vi "XL320_Reset.vi"(8 "Error In (no error)":errorcluster, 9 "Delay After Reset (2000 ms)":u32=2000, 10 "Motor ID (0)":u8, 11 "VISA resource name":refnum<visa-resource-name>) -> (0 "error out":errorcluster, 2 "Command to Serial":string, 3 "VISA resource name out":refnum<visa-resource-name>)   [LabVIEW 2017, in "Dynamixel XL320.lvlib"]
doc: "Resets the motor and to its default values. The motor ID will be 1 and the baud rate will be 57600 bps."
uses:
  <instrlib>/Dynamixel XL320 (Drivers instrument)/Dynamixel XL320.lvlib
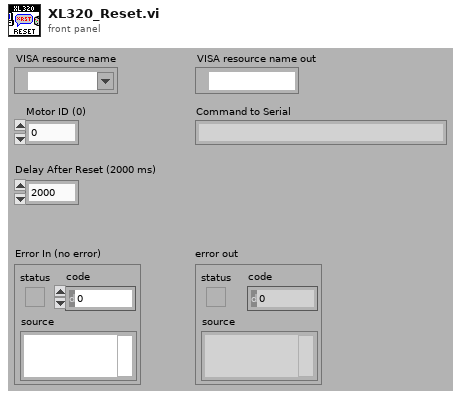
[diagram p1: front panel]
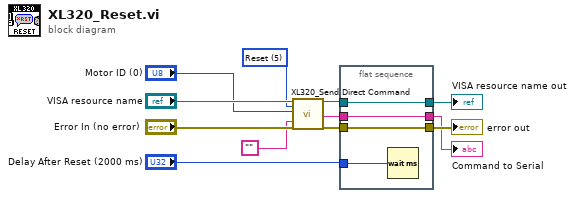
[diagram p0: block diagram]
diagram:
  w5 = u16 5 items=["Ping", "Read", "Write", "Registered Write", "Action", "Reset", "Sync Write"] ("Select Action")
  n1 = call <instrlib>:"XL320_Send Direct Command.vi"("VISA resource name"="VISA resource name", "Select Action"=w5, "Motor ID (0)"="Motor ID (0)", "Parameters"="", "Error in (no error)"="Error In (no error)") -> ("VISA resource name out"=w8:refnum<visa-resource-name>, "Command to Serial"=w2:string, "Error out"=w7:errorcluster)  [unwired: 12 in]
  n2 = flat-sequence {
    tunnel: "Delay After Reset (2000 ms)" -> [w16]
    tunnel: w7 -> [w13]
    tunnel: [w13] -> w11
    tunnel: w8 -> [w15]
    tunnel: [w15] -> w10
    tunnel: w2 -> [w14]
    tunnel: [w14] -> w1
    frame #0 {
      n3 = Wait (ms)(milliseconds to wait=w16) -> ()  [unwired: 1 out]
    }
  }
  "error out" <- w11
  "VISA resource name out" <- w10
  "Command to Serial" <- w1
